vi "get32bitInteger.vi"() -> (3 "outI32":i32)   [LabVIEW 2014]
uses:
  GlobalVariables.vi
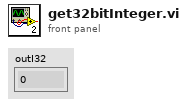
[diagram p1: front panel]
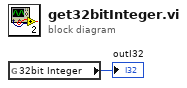
[diagram p0: block diagram]
diagram:
  n1 = global read "GlobalVariables.vi" "32bit Integer"() -> (→"outI32":i32)
